vi "CRYCompare file names.vi"(5 "data format":u16, 7 "save":enum16{"Data", "Results", "Waveforms"}(ring), 8 "Always replace":bool, 9 "Autosave folder":path, 10 "File name":string) -> (1 "Cancelled?":bool, 2 "Replace?":bool, 3 "File name  out":string)   [LabVIEW 2013]
uses:
  Data/CRYData & result stacks global.vi
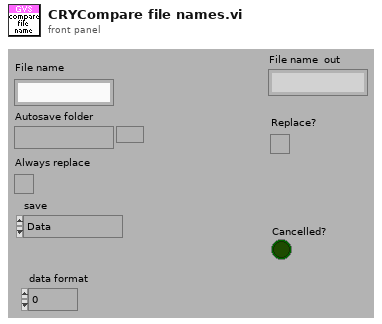
[diagram p1: front panel]
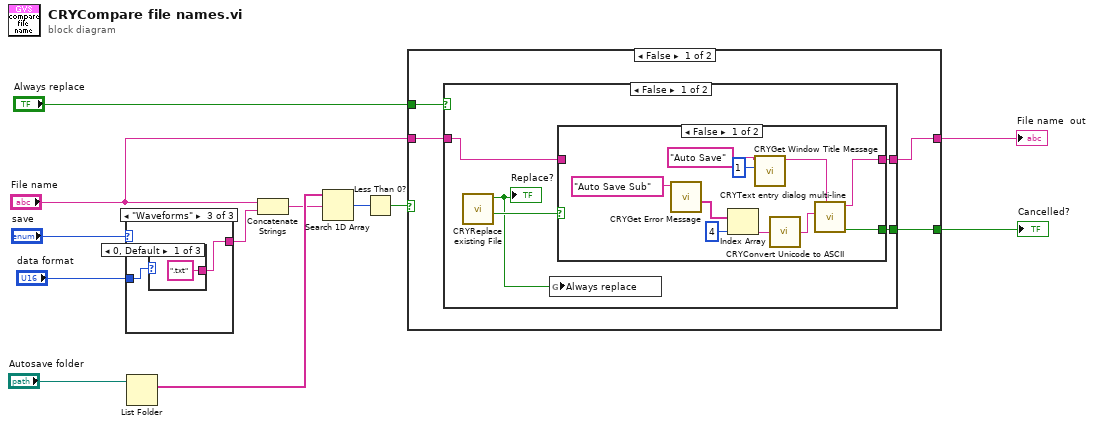
[diagram p0: block diagram]
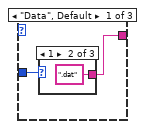
[diagram p2: hidden frame]
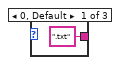
[diagram p3: hidden frame]
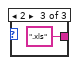
[diagram p4: hidden frame]
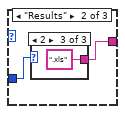
[diagram p5: hidden frame]
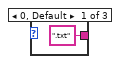
[diagram p6: hidden frame]
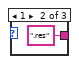
[diagram p7: hidden frame]
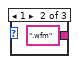
[diagram p8: hidden frame]
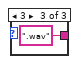
[diagram p9: hidden frame]
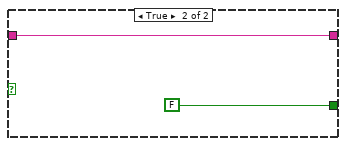
[diagram p10: hidden frame]
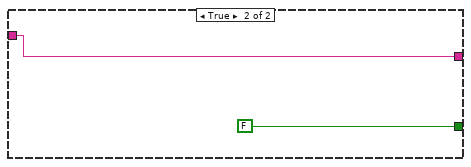
[diagram p11: hidden frame]
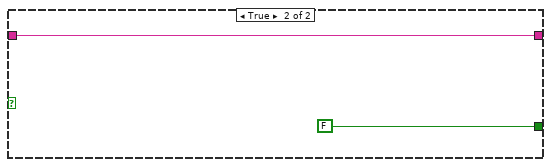
[diagram p12: hidden frame]
diagram:
  n1 = case shown="\"Waveforms\"" "save" {
    tunnel: [w14 w19 w23] -> w5
    tunnel: "data format" -> [w13 w18 w24]
    frame "Data", Default {
      n2 = case shown="1" w13 {
        tunnel: [".txt" ".dat" ".xls"] -> w14
        frame 0, Default {
        }
        frame 1 {
        }
        frame 2 {
        }
      }
    }
    frame "Results" {
      n3 = case shown="2" w18 {
        tunnel: [".txt" ".res" ".xls"] -> w19
        frame 0, Default {
        }
        frame 1 {
        }
        frame 2 {
        }
      }
    }
    frame "Waveforms" {
      n4 = case shown="0, Default" w24 {
        tunnel: [".txt" ".wfm" ".wav"] -> w23
        frame 0, Default {
        }
        frame 1 {
        }
        frame 3 {
        }
      }
    }
  }
  n5 = List Folder(path="Autosave folder") -> (filenames=w11:string[])  [unwired: 3 in, 3 out]
  n6 = Concatenate Strings("File name", w5) -> (w4:string)
  n7 = Search 1D Array(1D array=w11, element=w4) -> (index of element=w3:i32)  [unwired: 1 in]
  n8 = Less Than 0?(x=w3) -> (x < 0?=w10:bool)
  n9 = case shown="False" w10 {
    tunnel: "File name" -> [w31 w52]
    tunnel: [w30 w52] -> w8
    tunnel: "Always replace" -> [w29 _]
    tunnel: [w28 FALSE ("Cancelled?")] -> w6
    frame False {
      n10 = case shown="False" w29 {
        tunnel: w31 -> [w35 w50]
        tunnel: [w34 w50] -> w30
        tunnel: [w33 FALSE ("Cancelled?")] -> w28
        frame False {
          n11 = call "CRYReplace existing File.vi"() -> ("Yes or New?"=w36:bool, "Replace?"=w32:bool)  [unwired: 10 in]
          "Replace?" <- w32
          n12 = global write "CRYData & result stacks global.vi" "Always replace"(w32) -> ()
          n13 = case shown="False" w36 {
            tunnel: w35 -> [_ w48]
            tunnel: [w46 w48] -> w34
            tunnel: [w45 FALSE ("Cancelled?")] -> w33
            frame False {
              n14 = call "CRYGet Error Message.vi"("Kind"="Auto Save Sub") -> ("Unicode Message Sub"=w43:string[])  [unwired: 5 in, 5 out]
              n15 = Index Array(array=w43, index=4 ("Error No")) -> (element=w37:string)
              n16 = call "CRYGet Window Title Message.vi"("No"=1, "Kind"="Auto Save") -> ("Multibyte String"=w39:string)  [unwired: 4 in, 5 out]
              n17 = call "CRYConvert Unicode to ASCII.vi"("Unicode"=w37) -> ("ASCII"=w38:string)  [unwired: 4 in]
              n18 = call "CRYText entry dialog multi-line.vi"("Text"=w38, "Title Name"=w39) -> ("text entered"=w46:string, "Cancelled?"=w45:bool)  [unwired: 7 in]
            }
            frame True {
            }
          }
        }
        frame True {
        }
      }
    }
    frame True {
    }
  }
  "File name  out" <- w8
  "Cancelled?" <- w6
